vi "Configure Trace Buffer.vi"(4 "Buffer Time Stamp Format (0: Absolute)":i32(ring) items=["Absolute", "Delta"], 5 "Enable Buffer (0: Disable)":bool, 6 "Buffer Source (0: Raw Input Readings)":u16(ring) items=["Raw Input Readings", "CALC1 Readings", "CALC2 Readings"], 7 "Buffer Elements (CHAN,TST)":string="CHAN,TST", 8 "error in (no error)":errorcluster, 9 "Enable Auto Buffer Sizing (F: Disable)":bool, 10 "Buffer Size (100)":dbl=100.0, 11 "VISA resource name":refnum<visa-resource-name>) -> (0 "error out":errorcluster, 3 "VISA resource name out":refnum<visa-resource-name>)   [LabVIEW 2019, in "Keithley 6517.lvlib"]
doc: "Configures the auto buffer sizing, buffer size, and buffer elements."
uses:
  Keithley 6517.lvlib
panel:
  # "Models 6517A, 6517B Settings"
  # "Model 6514 Settings"
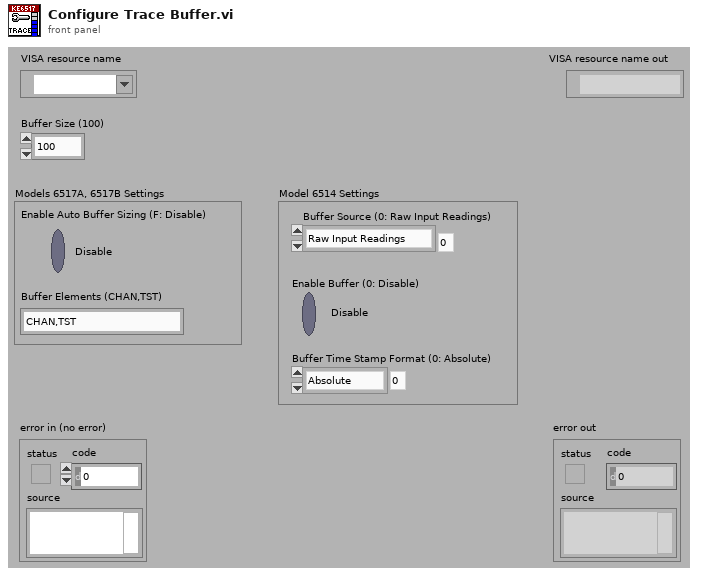
[diagram p1: front panel]
types:
  T1 = typedef "Keithley 6517.lvlib/Extended User Data.ctl" = cluster{"Instrument Model":i32}
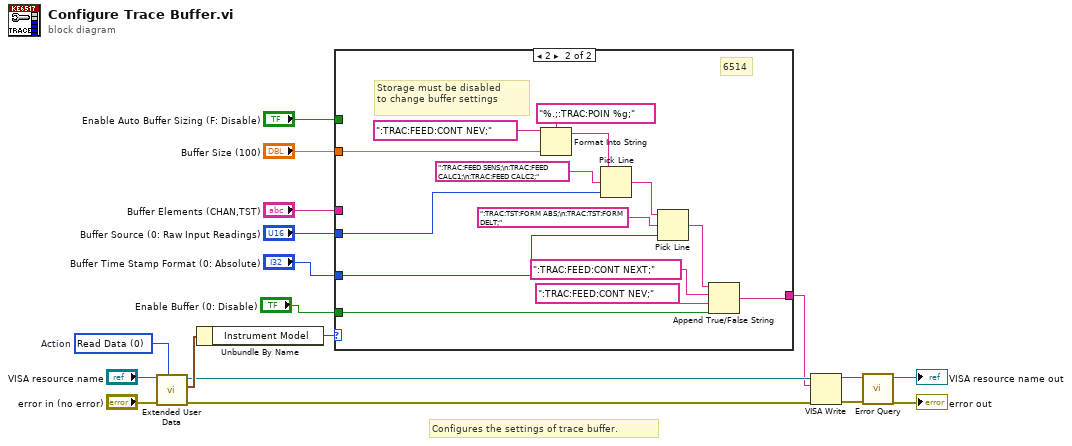
[diagram p0: block diagram]
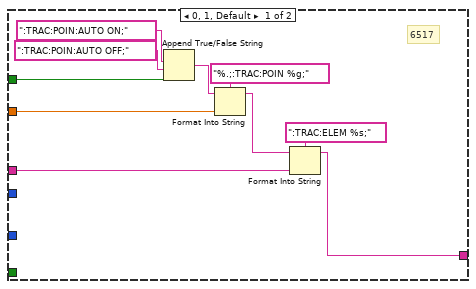
[diagram p2: hidden frame]
diagram:
  w9 = u16 0 items=["Read Data", "Write Data", "Clear Data", "Clear ALL Data"]  # Action
  # "Configures the settings of trace buffer."
  n1 = call "Extended User Data.vi"("Action (0: Read Data)"=w9, "error in (no error)"="error in (no error)", "VISA resource name"="VISA resource name") -> ("error out"=w6:errorcluster, "User Data Out"=w8:T1, "VISA resource name out"=w5:refnum<visa-resource-name>)  [unwired: 6 in]
  n2 = Unbundle By Name(w8) -> ("Instrument Model"=w7:i32)
  n3 = case shown="2" w7 {
    tunnel: "Enable Auto Buffer Sizing (F: Disable)" -> [w28 _]
    tunnel: "Buffer Size (100)" -> [w23 w41]
    tunnel: "Buffer Elements (CHAN,TST)" -> [w20 _]
    tunnel: "Buffer Source (0: Raw Input Readings)" -> [_ w40]
    tunnel: [w19 w31] -> w3
    tunnel: "Buffer Time Stamp Format (0: Absolute)" -> [_ w36]
    tunnel: "Enable Buffer (0: Disable)" -> [_ w33]
    frame 0, 1, Default {
      # "6517"
      n4 = Append True/False String(1:w28, 2:":TRAC:POIN:AUTO OFF;", 3:":TRAC:POIN:AUTO ON;") -> (0:w25:string)  [unwired: 1 in]
      n5 = Format Into String(format string="%.;:TRAC:POIN %g;", initial string=w25, w23) -> (resulting string=w22:string)  [unwired: 1 in, 1 out]
      n6 = Format Into String(format string=":TRAC:ELEM %s;", initial string=w22, w20) -> (resulting string=w19:string)  [unwired: 1 in, 1 out]
    }
    frame 2 {
      # "Storage must be disabled\nto change buffer settings"
      # "6514"
      n7 = Format Into String(format string="%.;:TRAC:POIN %g;", initial string=":TRAC:FEED:CONT NEV;" ("true string"), w41) -> (resulting string=w30:string)  [unwired: 1 in, 1 out]
      n8 = Pick Line(string ("")=w30, multi-line string=":TRAC:FEED SENS;\n:TRAC:FEED CALC1;\n:TRAC:FEED CALC2;", line index=w40) -> (output string=w37:string)
      n9 = Pick Line(string ("")=w37, multi-line string=":TRAC:TST:FORM ABS;\n:TRAC:TST:FORM DELT;", line index=w36) -> (output string=w32:string)
      n10 = Append True/False String(1:w33, 2:":TRAC:FEED:CONT NEV;" ("true string"), 3:":TRAC:FEED:CONT NEXT;" ("true string"), 4:w32) -> (0:w31:string)
    }
  }
  n11 = VISA Write(VISA resource name=w5, write buffer=w3, error in (no error)=w6) -> (VISA resource name out=w15:refnum<visa-resource-name>, error out=w14:errorcluster)  [unwired: 1 out]
  n12 = call "Error Query.vi"("error in (no error)"=w14, "VISA resource name"=w15) -> ("error out"=→"error out":errorcluster, "VISA resource name out"=→"VISA resource name out":refnum<visa-resource-name>)  [unwired: 6 in, 2 out]
